vi "Create.vi"(8 "error in (no error)":errorcluster caption="错误输入（无错误）") -> (0 "error out":errorcluster caption="错误输出", 3 "Color 输出":refnum<class "Color.lvclass"> caption="DNL_LabVIEW Object out")   [LabVIEW 2012, in "Color.lvclass"]
uses:
  Color.lvclass
  Color.lvclass/Color.ctl
  System.Drawing
panel:
  in  "Color 输入":refnum<class "Color.lvclass"> caption="DNL_LabVIEW Object in"
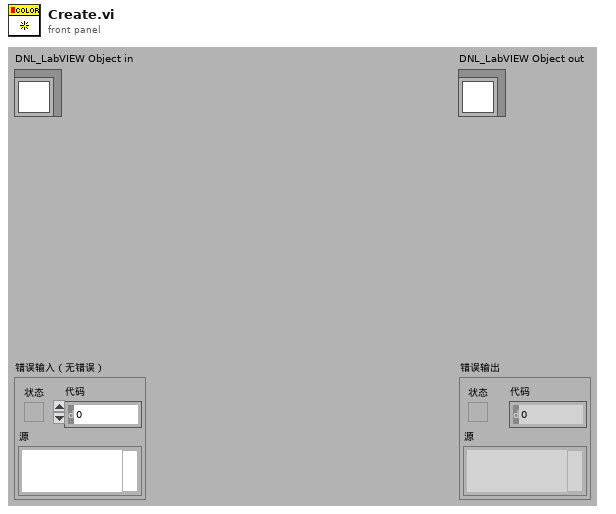
[diagram p1: front panel]
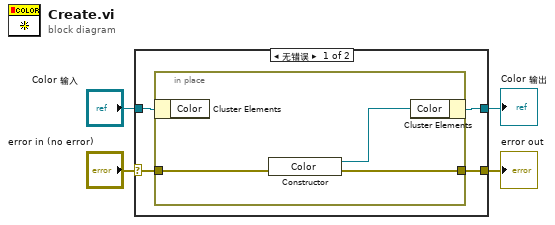
[diagram p0: block diagram]
diagram:
  n1 = case shown="无错误" "error in (no error)" {
    selector: "error in (no error)" -> [w7 w13]
    tunnel: [w5 w13] -> w3
    tunnel: [w6 w12] -> w1
    tunnel: "Color 输入" -> [w8 w12]
    frame No Error {
      n2 = in-place {
        in-place-border: w7 -> [w10]
        in-place-border: [w9] -> w5
        n3 = in-place-cluster #1(w8) -> ()  [unwired: 1 out]
        n4 = constructor class="Color"(error in=w10) -> (reference out=w11:refnum<k24>, error out=w9:errorcluster)  [unwired: 2 in, 1 out]
        n5 = in-place-cluster #1("Color"=w11) -> (w6:refnum<class "Color.lvclass">)
      }
    }
    frame Error {
    }
  }
  "error out" <- w3
  "Color 输出" <- w1
